vi "HEWH Water Density.vi"(8 "Error In":errorcluster, 11 "Input Temperature (°F)":dbl) -> (0 "Error Out":errorcluster, 3 "Density (lbm/gal)":dbl)   [LabVIEW 2016]
uses:
  <vilib>/Analysis/NI_AALPro.lvlib
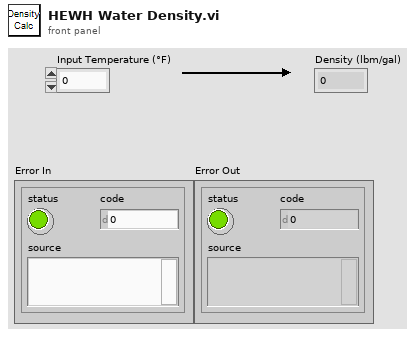
[diagram p1: front panel]
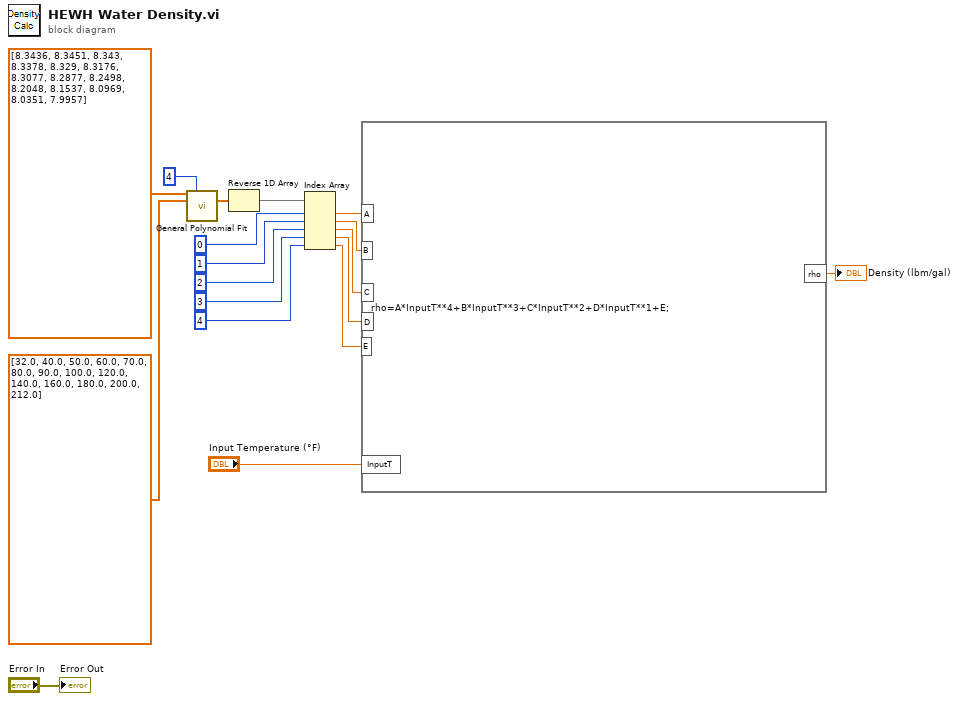
[diagram p0: block diagram]
diagram:
  n1 = call <vilib>:"General Polynomial Fit.vi"("Y"=dbl[] [8.3436, 8.3451, 8.343, 8.3378, 8.329, 8.3176, 8.3077, 8.2877, 8.2498, 8.2048, 8.1537, 8.0969, 8.0351, 7.9957], "polynomial order"=4, "X"=dbl[] [32.0, 40.0, 50.0, 60.0, 70.0, 80.0, 90.0, 100.0, 120.0, 140.0, 160.0, 180.0, 200.0, 212.0]) -> ("Polynomial Coefficients"=w14:dbl[])  [unwired: 9 in, 3 out]
  n2 = Reverse 1D Array(array=w14) -> (reversed array=w13:dbl[])
  n3 = Index Array(array=w13, index #1=0 ("index"), index #2=1 ("index"), index #3=2 ("index"), index #4=3 ("index"), index #5=4 ("index")) -> (element #1=w8:dbl, element #2=w7:dbl, element #3=w6:dbl, element #4=w5:dbl, element #5=w2:dbl)
  n4 = formula code="rho=A*InputT**4+B*InputT**3+C*InputT**2+D*InputT**1+E;"("A"=w8, "B"=w7, "C"=w6, "D"=w5, "InputT"="Input Temperature (°F)", "E"=w2) -> ("rho"=→"Density (lbm/gal)":dbl)
  "Error Out" <- "Error In"
